vi "DB UI Record Access.vi"(8 "error in":errorcluster) -> (0 "error out":errorcluster)   [LabVIEW 2017, in "Database.lvlib"]
doc: "Interface to accesss database"
uses:
  Database.lvlib
  Private Controls/Database Record.ctl
panel:
  out "Database Record out":T1
  in  "client":string
  in  "Task":enum16{"update record", "read record"}(ring)
  in  "Database Record":T1
  in  "stop":bool
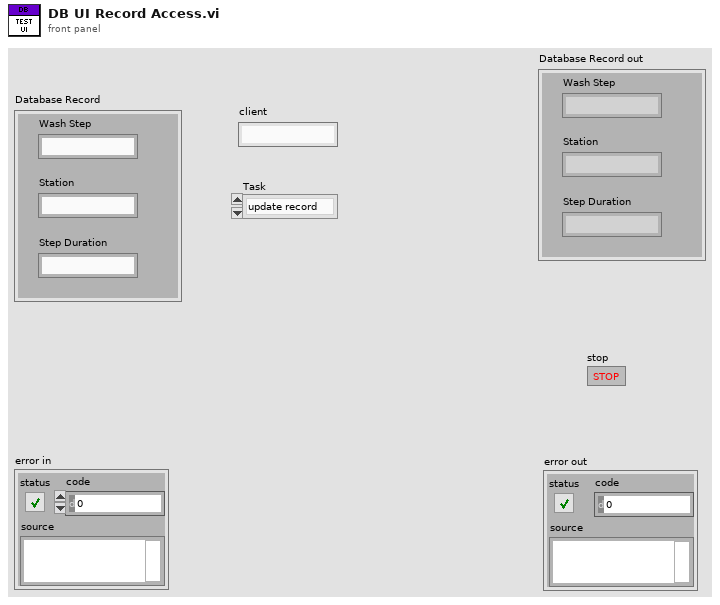
[diagram p1: front panel]
types:
  T1 = typedef "Database.lvlib/Database Record.ctl" = cluster{"Step Duration":string, "Station":string, "Wash Step":string}
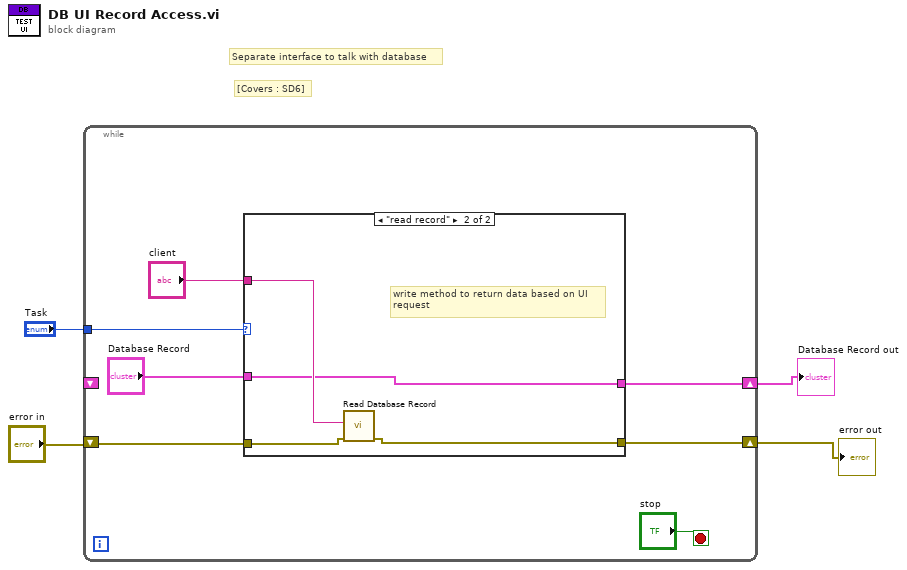
[diagram p0: block diagram]
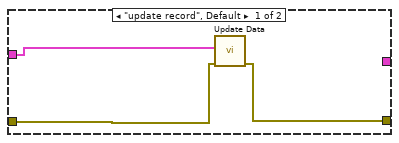
[diagram p2: hidden frame]
diagram:
  # "[Covers : SD6]"
  # "Separate interface to talk with database"
  n1 = while {
    tunnel: "Task" -> [w9]
    shift-right: [w7] -> w3
    shift-left: _ -> [_]
    shift-right: [w5] -> w1
    shift-left: "error in" -> [w6]
    stop <- "stop" stop-if-true
    n2 = case shown="\"read record\"" w9 {
      tunnel: "Database Record" -> [w12 w17]
      tunnel: "client" -> [_ w18]
      tunnel: [_ w17] -> w7
      tunnel: w6 -> [w14 w16]
      tunnel: [w13 w15] -> w5
      frame "update record", Default {
        n3 = call "Update Data.vi"("error in"=w14, "data"=w12) -> ("error out"=w13:errorcluster)  [unwired: 9 in]
      }
      frame "read record" {
        # "write method to return data based on UI\nrequest"
        n4 = call "Read Database Record.vi"("error in"=w16, "data"=w18) -> ("error out"=w15:errorcluster)  [unwired: 9 in]
      }
    }
  }
  "Database Record out" <- w3
  "error out" <- w1
